vi "globalSetUp.vi"(8 "error in":errorcluster, 11 "Deployment in":refnum<class "Deployment.lvclass">) -> (0 "error out":errorcluster, 3 "Deployment out":refnum<class "Deployment.lvclass">)   [LabVIEW 2020, in "Deployment.lvclass"]
uses:
  Deployment.lvclass
  <vilib>/NI/VeriStand Custom Device Testing Tools/VeriStandTestUtilities/VeriStandTestUtilities.lvlib
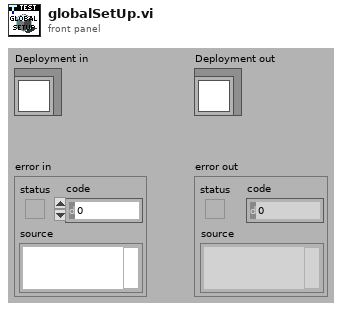
[diagram p1: front panel]
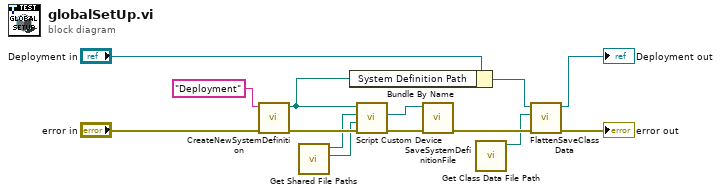
[diagram p0: block diagram]
diagram:
  n1 = call <vilib>:"CreateNewSystemDefinition.vi"("error in"="error in", "System Definition Name"="Deployment" ("Channel")) -> ("error out"=w12:errorcluster, "System Definition Path"=w7:path)  [unwired: 8 in]
  n2 = call "Get Shared File Paths.vi"() -> ("Hardware File"=w1:path, "Parameters File"=w2:path)  [unwired: 10 in]
  n3 = Bundle By Name(cluster="Deployment in", "System Definition Path"=w7) -> (w8:refnum<class "Deployment.lvclass">)
  n4 = call "Script Custom Device.vi"("error in"=w12, "Hardware Configuration File Path"=w1, "Parameters Configuration File Path"=w2, "System Definition File Path In"=w7) -> ("error out"=w14:errorcluster, "System Definition Reference"=w10:refnum<k24>)  [unwired: 4 in, 2 out]
  n5 = call <vilib>:"SaveSystemDefinitionFile.vi"("error in (no error)"=w14, "System Definition Reference in"=w10) -> ("error out"=w11:errorcluster)  [unwired: 8 in, 1 out]
  n6 = call "Get Class Data File Path.vi"() -> ("Class Data File Path"=w9:path)  [unwired: 11 in]
  n7 = call-dynamic "FlattenSaveClassData.vi"("error in"=w11, "Class Data File Path"=w9, "VeriStandTestCase in"=w8) -> ("error out"=→"error out":errorcluster, "VeriStandTestCase out"=→"Deployment out":refnum<class "Deployment.lvclass">)  [unwired: 7 in]
